vi "Keithley1b_2303_Measure.vi"(11 "YTESTER测试数据":T1) -> (3 "YTESTER结论":T2)   [LabVIEW 2017]
uses:
  YtCommon.lvlibp/yt`Step StepBaseInput.ctl
  YtCommon.lvlibp/yt`Step StepResult.ctl
  YtCommon.lvlibp/yt`Step TestData.ctl
  YtCommon.lvlibp/yt`Step System Queue.ctl
  Step`s VIs/YYLLGeneric/variable_W.ctl
  YtCommon.lvlibp/yt`Data-Ytester Type Data.ctl
  9150de1b-0d61-4f50-a2d9-e951e3cd4c84.vi
  72809a81-3210-4b0c-bdb6-030d0c0b3372.vi
  <vilib>/Analysis/baseanly.llb/Mean (DBL).vi
  19c99330-e7c4-4d8c-a522-00652d01c55d.vi
  c0565ce8-7c5d-4f1e-8a1f-5b5f61a1f71e.vi
  YtCommon.lvlibp
  <vilib>/Analysis/NI_AALBase.lvlib
panel:
  out "测量电流mA":dbl format="%#_12f"
  out "测量电压V":dbl format="%#_12f"
  in  "YTESTER开放参数":T4={"YTESTER_BaseInput"={"isTest"=FALSE, "isSkip"=FALSE, "StepName"="Keithley2303测量", "OnPass"=enum."Next", "OnFail"=enum."Next", "ReTestNumber"=0.0}, "VISA resource"="", "测试方式"=enum."测量N次取平均", "N次数"=1, "测量超时（s）"=10.0, "电压补偿（V）"=0.0, "电流补偿（mA）"=0.0, "测电流取绝对值？"=FALSE, "电压阈值上限（V）"=5.0, "电压阈值下限（V）"=0.0, "电流阈值上限（mA）"=50.0, "电流阈值下限（mA）"=1.0, "测量电压到变量(自定义建议#开头)"="不到变量", "测量电流到变量(自定义建议#开头)"="不到变量"}
  # "2303"
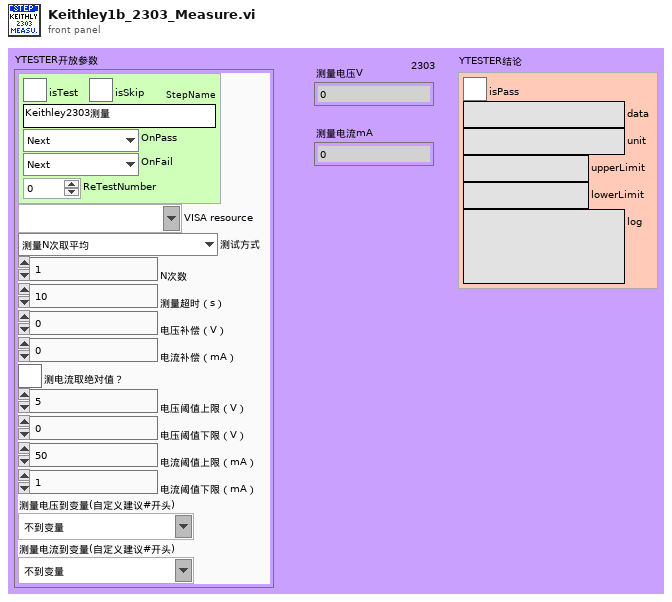
[diagram p1: front panel]
types:
  T1 = typedef "YtCommon.lvlibp/yt`Step TestData.ctl" = cluster{"Socket(From1)":i32, "SN":refnum<notifier>, "StopFlagRef":refnum<notifier>, "YT System Queue":refnum<queue>}
  T2 = typedef "YtCommon.lvlibp/yt`Step StepResult.ctl" = cluster{"isPass":bool, "data":string, "unit":string, "upperLimit":string, "lowerLimit":string, "log":string}
  T3 = typedef "YtCommon.lvlibp/yt`Step StepBaseInput.ctl" = cluster{"isTest":bool, "isSkip":bool, "StepName":string, "OnPass":enum16{"Next", "ToOVER", "Terminate"}, "OnFail":enum16{"Next", "ToOVER", "Terminate"}, "ReTestNumber":dbl}
  T4 = cluster{"YTESTER_BaseInput":T3, "VISA resource":refnum<visa-resource-name>, "测试方式":enum16{"测量N次取平均", "满足N次阈值取平均"}, "N次数":u8, "测量超时（s）":dbl, "电压补偿（V）":dbl, "电流补偿（mA）":dbl, "测电流取绝对值？":bool, "电压阈值上限（V）":dbl, "电压阈值下限（V）":dbl, "电流阈值上限（mA）":dbl, "电流阈值下限（mA）":dbl, "测量电压到变量(自定义建议#开头)":string, "测量电流到变量(自定义建议#开头)":string}
  T5 = typedef "variable_W.ctl" = cluster{"YT_TYPE":T6, "TypeData":string[], "Tips":string}
  T6 = typedef "YtCommon.lvlibp/yt`Data-Ytester Type Data.ctl" = enum16{"NULL", "NUM", "BOOL", "TXT", "ENUM", "TIME", "PATH", "VISA", "COMBO", "ColorBox", "RadioBtn", "Array_NUM", "Array_BOOL", "Array_TXT", "Array_ENUM", "Array_PATH", "Array_COMBO"}
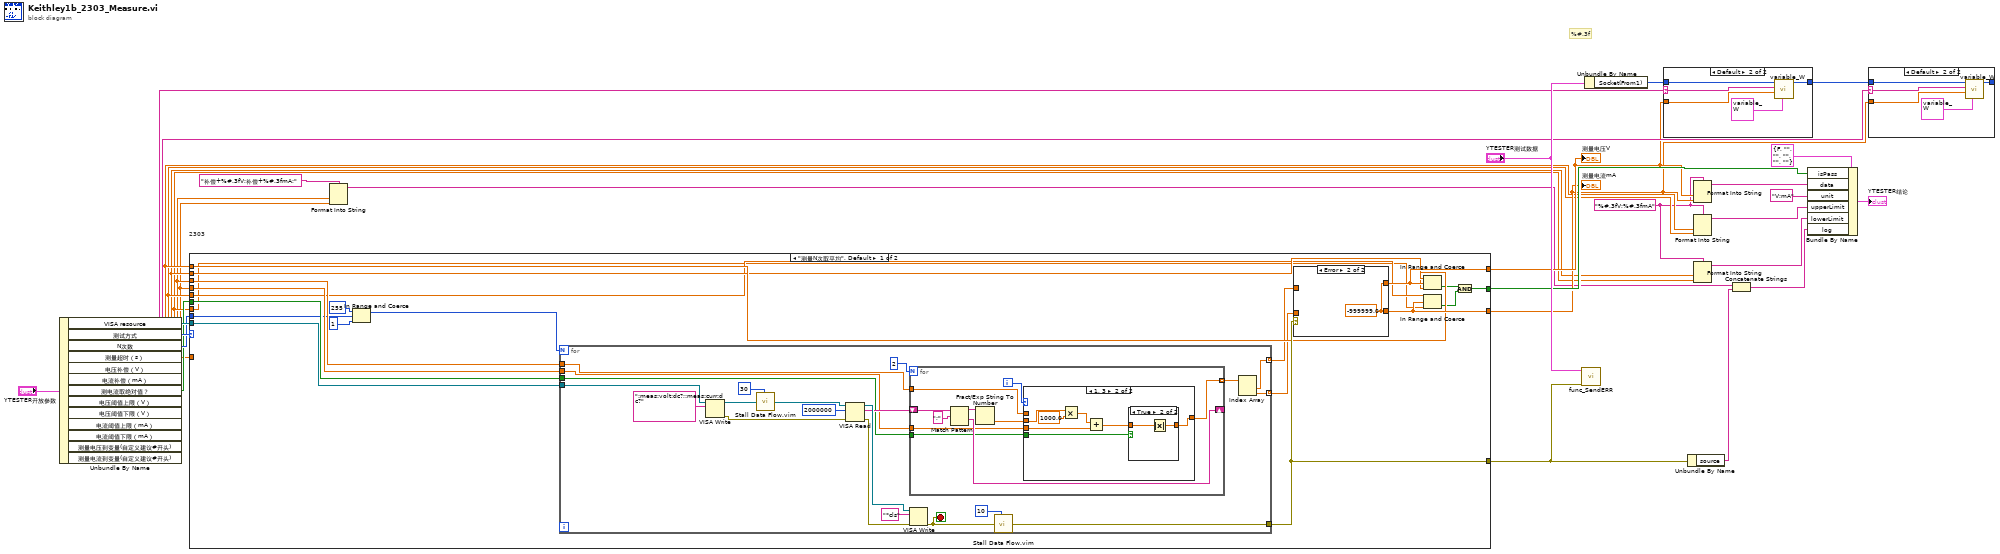
[diagram p0: block diagram]
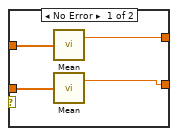
[diagram p4: hidden frame]
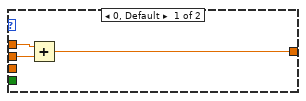
[diagram p5: hidden frame]
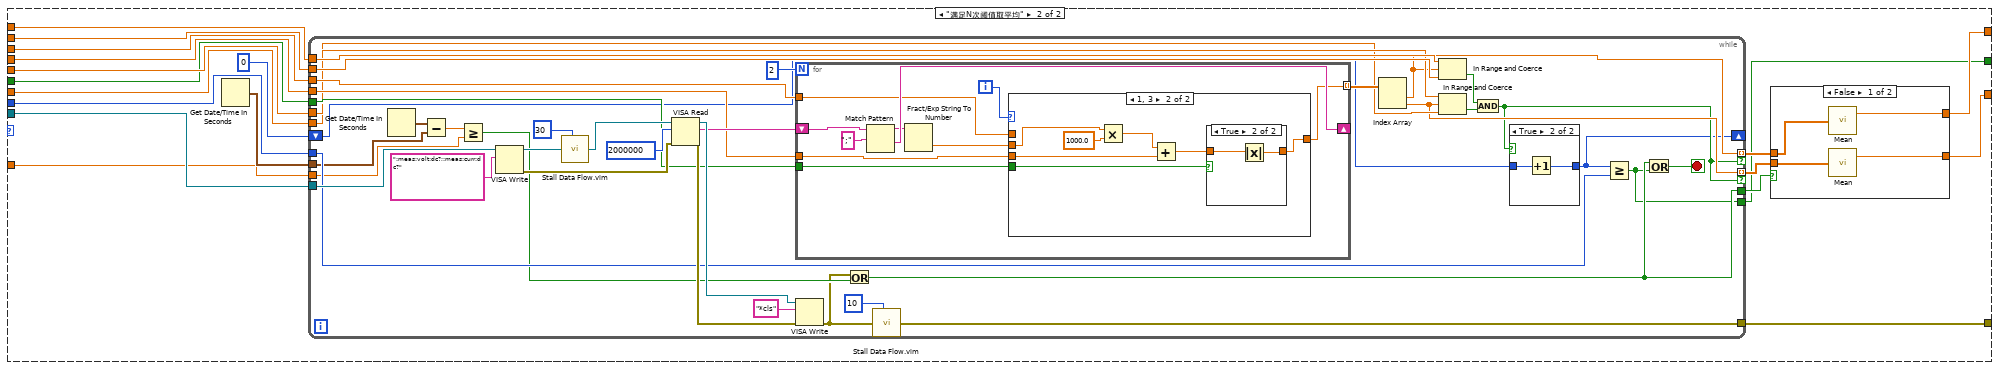
[diagram p7: hidden frame]
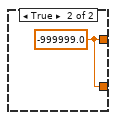
[diagram p8: hidden frame]
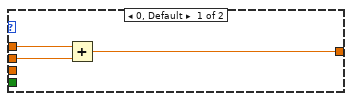
[diagram p10: hidden frame]
diagram:
  w8 = "%#.3fV;%#.3fmA" ("format string")
  # "%#.3f"
  n1 = Unbundle By Name("YTESTER开放参数") -> ("VISA resource"=w29:refnum<visa-resource-name>, "测试方式"=w30:enum16{"测量N次取平均", "满足N次阈值取平均"}, "N次数"=w28:u8, "测量超时（s）"=w22:dbl, "电压补偿（V）"=w4:dbl, "电流补偿（mA）"=w3:dbl, "测电流取绝对值？"=w27:bool, "电压阈值上限（V）"=w12:dbl, "电压阈值下限（V）"=w10:dbl, "电流阈值上限（mA）"=w11:dbl, "电流阈值下限（mA）"=w9:dbl, "测量电压到变量(自定义建议#开头)"=w24:string, "测量电流到变量(自定义建议#开头)"=w23:string)
  n2 = case "2303" shown="\"测量N次取平均\", Default" w30 {
    tunnel: w29 -> [w52 w108]
    tunnel: w28 -> [w38 w107]
    tunnel: w27 -> [w51 w109]
    tunnel: w4 -> [w50 w111]
    tunnel: w3 -> [w49 w110]
    tunnel: [w48 w119] -> w17
    tunnel: [w47 w120] -> w18
    tunnel: w12 -> [w45 w118]
    tunnel: w10 -> [w44 w117]
    tunnel: w11 -> [w43 w116]
    tunnel: w9 -> [w42 w115]
    tunnel: w22 -> [_ w105]
    tunnel: [w46 w103] -> w7
    tunnel: [w41 w102] -> w19
    frame "测量N次取平均", Default {
      n3 = In Range and Coerce(upper limit=u8 255, x=w38, lower limit=u8 1) -> (coerced(x)=w37:u8)  [unwired: 1 out]
      n4 = for {
        N: w37 -> [_]
        tunnel: [w67] -> w36 mode=indexing
        tunnel: [w66] -> w35 mode=indexing
        tunnel: w52 -> [w65]
        tunnel: w51 -> [w64]
        tunnel: w50 -> [w63]
        tunnel: w49 -> [w62]
        tunnel: [w58] -> w46
        stop <- w59 stop-if-true
        n5 = VISA Write(VISA resource name=w65, write buffer=":meas:volt:dc?;:meas:curr:dc?") -> (VISA resource name out=w76:refnum<visa-resource-name>, error out=w74:errorcluster)  [unwired: 1 in, 1 out]
        n6 = call "Stall Data Flow.vim"("value in"=w76, "milliseconds to wait"=u32 30) -> ("value out"=w73:refnum<visa-resource-name>)  [unwired: 1 out]
        n7 = VISA Read(VISA resource name=w73, byte count=u32 2000000, error in (no error)=w74) -> (VISA resource name out=w77:refnum<visa-resource-name>, read buffer=w75:string, error out=w78:errorcluster)  [unwired: 1 out]
        n8 = for {
          N: 2 -> [_]
          shift-right: [w87] -> _
          shift-left: w75 -> [w88]
          tunnel: w64 -> [w82]
          tunnel: w63 -> [w81]
          tunnel: w62 -> [w80]
          tunnel: [w79] -> w61 mode=indexing
          i -> [w83]
          n9 = Match Pattern(string=w88, regular expression=";") -> (before substring=w85:string, after substring=w87:string)  [unwired: 1 in, 2 out]
          n10 = Fract/Exp String To Number(string=w85) -> (number=w84:dbl)  [unwired: 3 in, 1 out]
          n11 = case shown="1, 3" w83 {
            tunnel: w84 -> [w91 w98]
            tunnel: [w90 w95] -> w79
            tunnel: w82 -> [_ w96]
            tunnel: w81 -> [w89 _]
            tunnel: w80 -> [_ w92]
            frame 0, Default {
              n12 = Add(x=w89, y=w91) -> (x+y=w90:dbl)
            }
            frame 1, 3 {
              n13 = Multiply(x=w98, y=1000.0) -> (x*y=w94:dbl)
              n14 = Add(x=w94, y=w92) -> (x+y=w93:dbl)
              n15 = case shown="True" w96 {
                tunnel: [w99 w100] -> w95
                tunnel: w93 -> [w99 w101]
                frame False {
                }
                frame True {
                  n16 = Absolute Value(x=w101) -> (abs(x)=w100:dbl)
                }
              }
            }
          }
        }
        n17 = VISA Write(VISA resource name=w77, write buffer="*cls", error in (no error)=w78) -> (error out=w59:errorcluster)  [unwired: 2 out]
        n18 = call "Stall Data Flow.vim"("value in"=w59, "milliseconds to wait"=u32 10) -> ("value out"=w58:errorcluster)  [unwired: 1 out]
        n19 = Index Array(array=w61) -> (element #1=w67:dbl, element #2=w66:dbl)  [unwired: 2 in]
      }
      n20 = case shown="Error" w46 {
        tunnel: w36 -> [w56 _]
        tunnel: w35 -> [w55 _]
        tunnel: [w54 w57] -> w47
        tunnel: [w53 w57] -> w48
        frame No Error {
          n21 = call-poly <vilib>:"Mean.vi"("X"=w56) -> ("mean"=w54:dbl)  [unwired: 1 out]
          n22 = call-poly <vilib>:"Mean.vi"("X"=w55) -> ("mean"=w53:dbl)  [unwired: 1 out]
        }
        frame Error {
          w57 = -999999.0 ("mean")
        }
      }
      n23 = In Range and Coerce(upper limit=w45, x=w47, lower limit=w44) -> (In Range?=w33:bool)  [unwired: 1 out]
      n24 = In Range and Coerce(upper limit=w43, x=w48, lower limit=w42) -> (In Range?=w34:bool)  [unwired: 1 out]
      n25 = And(x=w33, y=w34) -> (x .and. y?=w41:bool)
    }
    frame "满足N次阈值取平均" {
      n26 = Get Date/Time In Seconds() -> (seconds since 1Jan1904=w106:timestamp)
      n27 = while {
        tunnel: [w142] -> w114 mode=indexing if=w139
        tunnel: [w141] -> w113 mode=indexing if=w139
        tunnel: w108 -> [w153]
        tunnel: w109 -> [w152]
        tunnel: w111 -> [w151]
        tunnel: w110 -> [w150]
        tunnel: w118 -> [w146]
        tunnel: w117 -> [w145]
        tunnel: w116 -> [w144]
        tunnel: w115 -> [w143]
        shift-right: [w130] -> _
        shift-left: u8 0 -> [w140]
        tunnel: w107 -> [w138]
        tunnel: w106 -> [w136]
        tunnel: w105 -> [w133]
        tunnel: [w131] -> w104
        tunnel: [w127] -> w103
        tunnel: [w129] -> w102
        stop <- w135 stop-if-true
        n28 = Get Date/Time In Seconds() -> (seconds since 1Jan1904=w137:timestamp)
        n29 = Subtract(x=w137, y=w136) -> (x-y=w134:dbl)
        n30 = Greater Or Equal?(x=w134, y=w133) -> (x >= y?=w132:bool)
        n31 = VISA Write(VISA resource name=w153, write buffer=":meas:volt:dc?;:meas:curr:dc?") -> (VISA resource name out=w162:refnum<visa-resource-name>, error out=w160:errorcluster)  [unwired: 1 in, 1 out]
        n32 = call "Stall Data Flow.vim"("value in"=w162, "milliseconds to wait"=u32 30) -> ("value out"=w159:refnum<visa-resource-name>)  [unwired: 1 out]
        n33 = VISA Read(VISA resource name=w159, byte count=u32 2000000, error in (no error)=w160) -> (VISA resource name out=w163:refnum<visa-resource-name>, read buffer=w161:string, error out=w164:errorcluster)  [unwired: 1 out]
        n34 = for {
          N: 2 -> [_]
          shift-right: [w176] -> _
          shift-left: w161 -> [w177]
          tunnel: w152 -> [w171]
          tunnel: w151 -> [w170]
          tunnel: w150 -> [w169]
          tunnel: [w168] -> w149 mode=indexing
          i -> [w172]
          n35 = Match Pattern(string=w177, regular expression=";") -> (before substring=w174:string, after substring=w176:string)  [unwired: 1 in, 2 out]
          n36 = Fract/Exp String To Number(string=w174) -> (number=w173:dbl)  [unwired: 3 in, 1 out]
          n37 = case shown="1, 3" w172 {
            tunnel: w173 -> [w180 w187]
            tunnel: [w179 w184] -> w168
            tunnel: w171 -> [_ w185]
            tunnel: w170 -> [w178 _]
            tunnel: w169 -> [_ w181]
            frame 0, Default {
              n38 = Add(x=w178, y=w180) -> (x+y=w179:dbl)
            }
            frame 1, 3 {
              n39 = Multiply(x=w187, y=1000.0) -> (x*y=w183:dbl)
              n40 = Add(x=w183, y=w181) -> (x+y=w182:dbl)
              n41 = case shown="True" w185 {
                tunnel: [w188 w189] -> w184
                tunnel: w182 -> [w188 w190]
                frame False {
                }
                frame True {
                  n42 = Absolute Value(x=w190) -> (abs(x)=w189:dbl)
                }
              }
            }
          }
        }
        n43 = VISA Write(VISA resource name=w163, write buffer="*cls", error in (no error)=w164) -> (error out=w128:errorcluster)  [unwired: 2 out]
        n44 = Or(x=w128, y=w132) -> (x .or. y?=w131:bool)
        n45 = call "Stall Data Flow.vim"("value in"=w128, "milliseconds to wait"=u32 10) -> ("value out"=w127:errorcluster)  [unwired: 1 out]
        n46 = Index Array(array=w149) -> (element #1=w142:dbl, element #2=w141:dbl)  [unwired: 2 in]
        n47 = In Range and Coerce(upper limit=w146, x=w142, lower limit=w145) -> (In Range?=w148:bool)  [unwired: 1 out]
        n48 = In Range and Coerce(upper limit=w144, x=w141, lower limit=w143) -> (In Range?=w147:bool)  [unwired: 1 out]
        n49 = And(x=w148, y=w147) -> (x .and. y?=w139:bool)
        n50 = case shown="True" w139 {
          tunnel: w140 -> [w165 w167]
          tunnel: [w165 w166] -> w130
          frame False {
          }
          frame True {
            n51 = Increment(x=w167) -> (x+1=w166:u8)
          }
        }
        n52 = Greater Or Equal?(x=w130, y=w138) -> (x >= y?=w129:bool)
        n53 = Or(x=w131, y=w129) -> (x .or. y?=w135:bool)
      }
      n54 = case shown="False" w104 {
        tunnel: [w124 w125] -> w120
        tunnel: [w123 w125] -> w119
        tunnel: w114 -> [w122 _]
        tunnel: w113 -> [w121 _]
        frame False {
          n55 = call-poly <vilib>:"Mean.vi"("X"=w122) -> ("mean"=w124:dbl)  [unwired: 1 out]
          n56 = call-poly <vilib>:"Mean.vi"("X"=w121) -> ("mean"=w123:dbl)  [unwired: 1 out]
        }
        frame True {
          w125 = -999999.0 ("mean")
        }
      }
    }
  }
  "测量电压V" <- w18
  "测量电流mA" <- w17
  n57 = Format Into String(format string="补偿+%#.3fV;补偿+%#.3fmA;", w4, w3) -> (resulting string=w1:string)  [unwired: 2 in, 1 out]
  n58 = call "func_SendERR.vi"("ERR (String\\Errclust)"=w7, "YTESTER测试数据 in"="YTESTER测试数据") -> ()  [unwired: 9 in, 1 out]
  n59 = Unbundle By Name("YTESTER测试数据") -> ("Socket(From1)"=w25:i32)
  n60 = case shown="Default" w24 {
    selector: w24 -> [_ w195]
    tunnel: w25 -> [w191 w196]
    tunnel: w18 -> [_ w193]
    tunnel: [w191 w192] -> w26
    frame "不到变量" {
    }
    frame Default {
      n61 = call "variable_W.vi"("附加的Information"=T5 {"YT_TYPE"=enum."NUM", "TypeData"=[], "Tips"="yt_Keithley电压测量缓存"}, "待写入池的输入控件"=w193, "待写入池变量名称"=w195, "函数池名称 in"=w196) -> ("函数池名称 out"=w192:i32)  [unwired: 5 in, 2 out]
    }
  }
  n62 = Unbundle By Name(w7) -> ("source"=w6:string)
  n63 = Format Into String(format string=w8, w18, w17) -> (resulting string=w16:string)  [unwired: 2 in, 1 out]
  n64 = Format Into String(format string=w8, w12, w11) -> (resulting string=w14:string)  [unwired: 2 in, 1 out]
  n65 = Format Into String(format string=w8, w10, w9) -> (resulting string=w13:string)  [unwired: 2 in, 1 out]
  n66 = Concatenate Strings(w1, w6) -> (w2:string)
  n67 = Bundle By Name(cluster=T2 {"isPass"=FALSE, "data"="", "unit"="", "upperLimit"="", "lowerLimit"="", "log"=""} ("Result"), "isPass"=w19, "data"=w16, "unit"="V;mA", "upperLimit"=w14, "lowerLimit"=w13, "log"=w2) -> (→"YTESTER结论":T2)
  n68 = case shown="Default" w23 {
    selector: w23 -> [_ w201]
    tunnel: w26 -> [w197 w202]
    tunnel: w17 -> [_ w199]
    tunnel: [w197 w198] -> _
    frame "不到变量" {
    }
    frame Default {
      n69 = call "variable_W.vi"("附加的Information"=T5 {"YT_TYPE"=enum."NUM", "TypeData"=[], "Tips"="yt_Keithley电流测量缓存"}, "待写入池的输入控件"=w199, "待写入池变量名称"=w201, "函数池名称 in"=w202) -> ("函数池名称 out"=w198:i32)  [unwired: 5 in, 2 out]
    }
  }
